vi "Register for Events.vi"(8 "error in (no error)":errorcluster, 11 "Stage State Data":refnum<data-value>) -> (0 "error out":errorcluster, 2 "Event Registration Refnum":refnum<event-registration>, 3 "Stage State Data":refnum<data-value>)   [LabVIEW 2022 SP3, in "XY Stage Data Class.lvclass"]
uses:
  XY Stage Data Class.lvclass
  XY Stage Data Class.lvclass/XY Stage Data Class.ctl
  XY Position.ctl
  Moving.ctl
  Homed.ctl
  Acceleration.ctl
  Current Speed.ctl
  Events.ctl
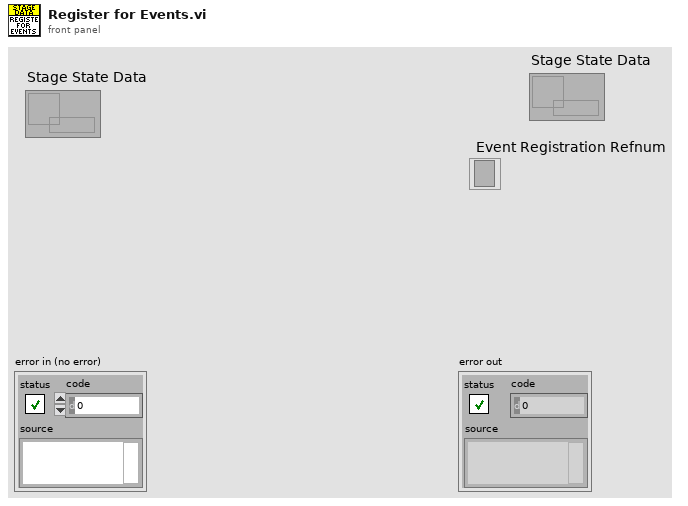
[diagram p1: front panel]
types:
  T1 = typedef "XY Stage Data Class.lvclass/Events.ctl" = cluster{"XY Position":refnum<user-event>, "Moving":refnum<user-event>, "Homed":refnum<user-event>, "Acceleration":refnum<user-event>, "Current Speed":refnum<user-event>}
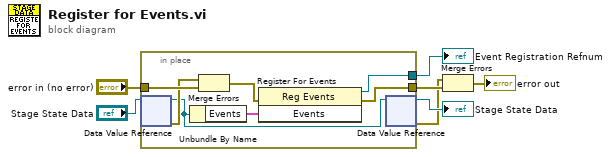
[diagram p0: block diagram]
diagram:
  n1 = in-place {
    in-place-border: "error in (no error)" -> [w13]
    in-place-border: [w12] -> w5
    in-place-border: [w11] -> w4
    n2 = in-place-dvr #1("Stage State Data") -> (w8:refnum<class "XY Stage Data Class.lvclass">, w9:errorcluster)
    n3 = Unbundle By Name(w8) -> ("Events"=w14:T1)
    n4 = Merge Errors(w9, w13) -> (w10:errorcluster)
    n5 = register-events(error in=w10, w14) -> (reference out=w11:refnum<event-registration>, error out=w12:errorcluster)  [unwired: 1 in]
    n6 = in-place-dvr #1(w8) -> (→"Stage State Data":refnum<data-value>, w1:errorcluster)
  }
  "Event Registration Refnum" <- w4
  n7 = Merge Errors(w1, w5) -> (→"error out":errorcluster)
